vi "Name_Sequence.vi"() -> (1 "SequenceName":string)   [LabVIEW 2016, in "SeqProcessor.lvlib"]
uses:
  SeqProcessor.lvlib
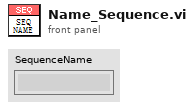
[diagram p1: front panel]
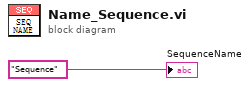
[diagram p0: block diagram]
diagram:
  "SequenceName" <- "Sequence" ("SequenceName")
